vi "racunanje_matrica.vi"(6 "dq2":dbl, 7 "g":dbl, 9 "dq1":dbl, 10 "q2":dbl, 11 "q1":dbl) -> (1 "M":T1, 2 "G":T1, 3 "C":T1)   [LabVIEW 2014]
uses:
  <vilib>/Analysis/Matrix/Datatypes/RealMatrix.ctl
  <vilib>/Analysis/Matrix/NI_Matrix.lvlib
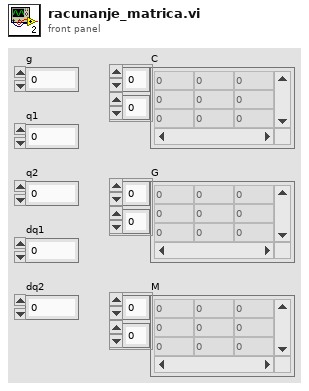
[diagram p1: front panel]
types:
  T1 = typedef "NI_Matrix.lvlib/RealMatrix.ctl" = dbl[][]
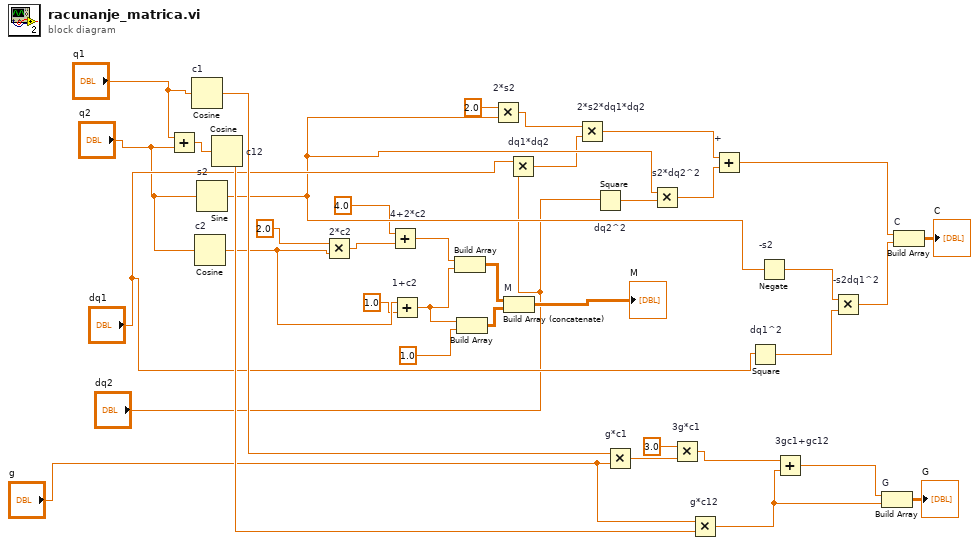
[diagram p0: block diagram]
diagram:
  n1 = Add(x="q1", y="q2") -> (x+y=w1:dbl)
  n2 = Cosine "c1"(x="q1") -> (cos(x)=w27:dbl)
  n3 = Cosine "c2"(x="q2") -> (cos(x)=w8:dbl)
  n4 = Sine "s2"(x="q2") -> (sin(x)=w21:dbl)
  n5 = Cosine "c12"(x=w1) -> (cos(x)=w32:dbl)
  n6 = Multiply "2*c2"(x=2.0, y=w8) -> (x*y=w5:dbl)
  n7 = Add "4+2*c2"(x=4.0, y=w5) -> (x+y=w9:dbl)
  n8 = Add "1+c2"(x=w8, y=1.0 ("x")) -> (x+y=w10:dbl)
  n9 = Build Array(w9, w10) -> (w12:T1)
  n10 = Build Array(w10, 1.0 ("x")) -> (w13:T1)
  n11 = Multiply "2*s2"(x=2.0, y=w21) -> (x*y=w15:dbl)
  n12 = Build Array (concatenate) "M"(w12, w13) -> (→"M":T1)
  n13 = Multiply "dq1*dq2"(x="dq1", y="dq2") -> (x*y=w16:dbl)
  n14 = Multiply "2*s2*dq1*dq2"(x=w15, y=w16) -> (x*y=w17:dbl)
  n15 = Square "dq2^2"(x="dq2") -> (x^2=w19:dbl)
  n16 = Multiply "g*c1"(x=w27, y="g") -> (x*y=w28:dbl)
  n17 = Multiply "s2*dq2^2"(x=w21, y=w19) -> (x*y=w20:dbl)
  n18 = Multiply "3g*c1"(x=3.0, y=w28) -> (x*y=w30:dbl)
  n19 = Multiply "g*c12"(x="g", y=w32) -> (x*y=w34:dbl)
  n20 = Add "+"(x=w17, y=w20) -> (x+y=w25:dbl)
  n21 = Square "dq1^2"(x="dq1") -> (x^2=w24:dbl)
  n22 = Negate "-s2"(x=w21) -> (-x=w23:dbl)
  n23 = Add "3gc1+gc12"(x=w30, y=w34) -> (x+y=w33:dbl)
  n24 = Multiply "-s2dq1^2"(x=w23, y=w24) -> (x*y=w26:dbl)
  n25 = Build Array "G"(w33, w34) -> (→"G":T1)
  n26 = Build Array "C"(w25, w26) -> (→"C":T1)
